vi "Get BooleanArray.vi"(8 "error in (no error)":errorcluster, 11 "BooleanArrayMsg in":refnum<class "BooleanArrayMsg.lvclass">) -> (0 "error out":errorcluster, 2 "Message Data":bool[](array[boolean]), 3 "BooleanArrayMsg out":refnum<class "BooleanArrayMsg.lvclass">)   [LabVIEW 2009, in "LapDog.Messaging.v2.NativeArrays.lvlib" / "BooleanArrayMsg.lvclass"]
doc: "Returns the data contained in the message.\n\nThis method executes regardless of the error in state."
uses:
  BooleanArrayMsg.lvclass
  BooleanArrayMsg.lvclass/BooleanArrayMsg.ctl
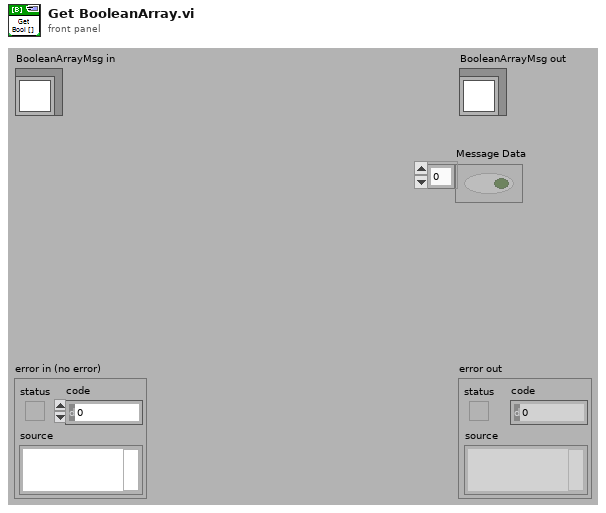
[diagram p1: front panel]
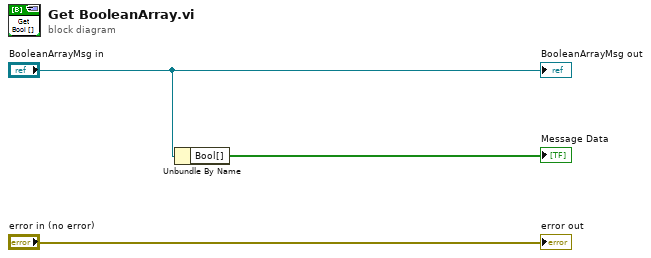
[diagram p0: block diagram]
diagram:
  n1 = Unbundle By Name("BooleanArrayMsg in") -> ("Bool[]"=→"Message Data":bool[])
  "error out" <- "error in (no error)"
  "BooleanArrayMsg out" <- "BooleanArrayMsg in"
